vi "创建参数二维码.vi"() -> ()   [LabVIEW 2016, in "wxpusher.lvlib"]
uses:
  wxpusher.lvlib
  System.Windows.Forms
  <vilib>/Utility/miscctls.llb/LVPointTypeDef.ctl
  <vilib>/httpClient/POSTBuffer.vi
  <vilib>/httpClient/LabVIEWHTTPClient.lvlib
panel:
  out "url":string
  out "data.uid":string
  in  "测试":bool
  out "关注时间":string
  in  "关注信息":refnum<k24>(container) caption="黎山萧"
  in  "关闭":bool
  in  "带参数二维码":refnum<k24>(container)
  out "error out":errorcluster caption="错误输出"
  in  "error in (no error)":errorcluster caption="错误输入（无错误）"
  # "请使用微信扫描以下二维码"
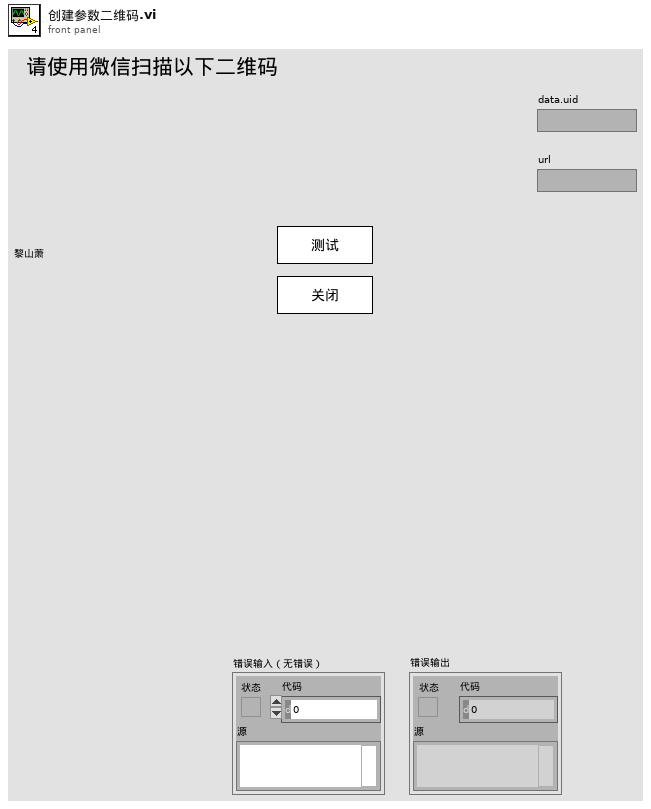
[diagram p1: front panel]
types:
  T1 = enum16{"初始化", "创建带参数二维码", "与服务器创建连接", "定时发送特征码", "接收回调信息", "处理回调信息", "展示关注信息", "结束"}[]
  T2 = enum16{"初始化", "创建带参数二维码", "与服务器创建连接", "定时发送特征码", "接收回调信息", "处理回调信息", "展示关注信息", "结束"}
  T3 = typedef "LVPointTypeDef.ctl" = cluster{"Horizontal":i16, "Vertical":i16}
  T4 = cluster{"code":u64, "msg":string, "data":cluster{"expires":u64, "code":string, "shortUrl":string, "extra":string, "url":string}, "success":bool}
  T5 = cluster{"appToken":string, "extra":string, "validTime":i32}
  T6 = enum16{"Standard", "Buffered", "CRLF", "Immediate"}
  T7 = cluster{"data":cluster{"action":string, "data":cluster{"appKey":string, "appName":string, "source":string, "time":u64, "uid":string, "userHeadImg":string, "userName":string, "extra":string}}}
  T8 = cluster{"cmd":string, "data":cluster{"png":u8[]}}
  T9 = typedef "LabVIEWHTTPClient.lvlib/ClientHandle.ctl" = refnum<k1>
  T10 = cluster{"expires":u64, "code":string, "shortUrl":string, "extra":string, "url":string}
  T11 = cluster{"action":string, "data":cluster{"appKey":string, "appName":string, "source":string, "time":u64, "uid":string, "userHeadImg":string, "userName":string, "extra":string}}
  T12 = cluster{"action":string, "data":cluster{"appKey":string, "appName":string, "source":string, "time":u64, "uid":string, "userHeadImg":string, "userName":string, "extra":string}}[]
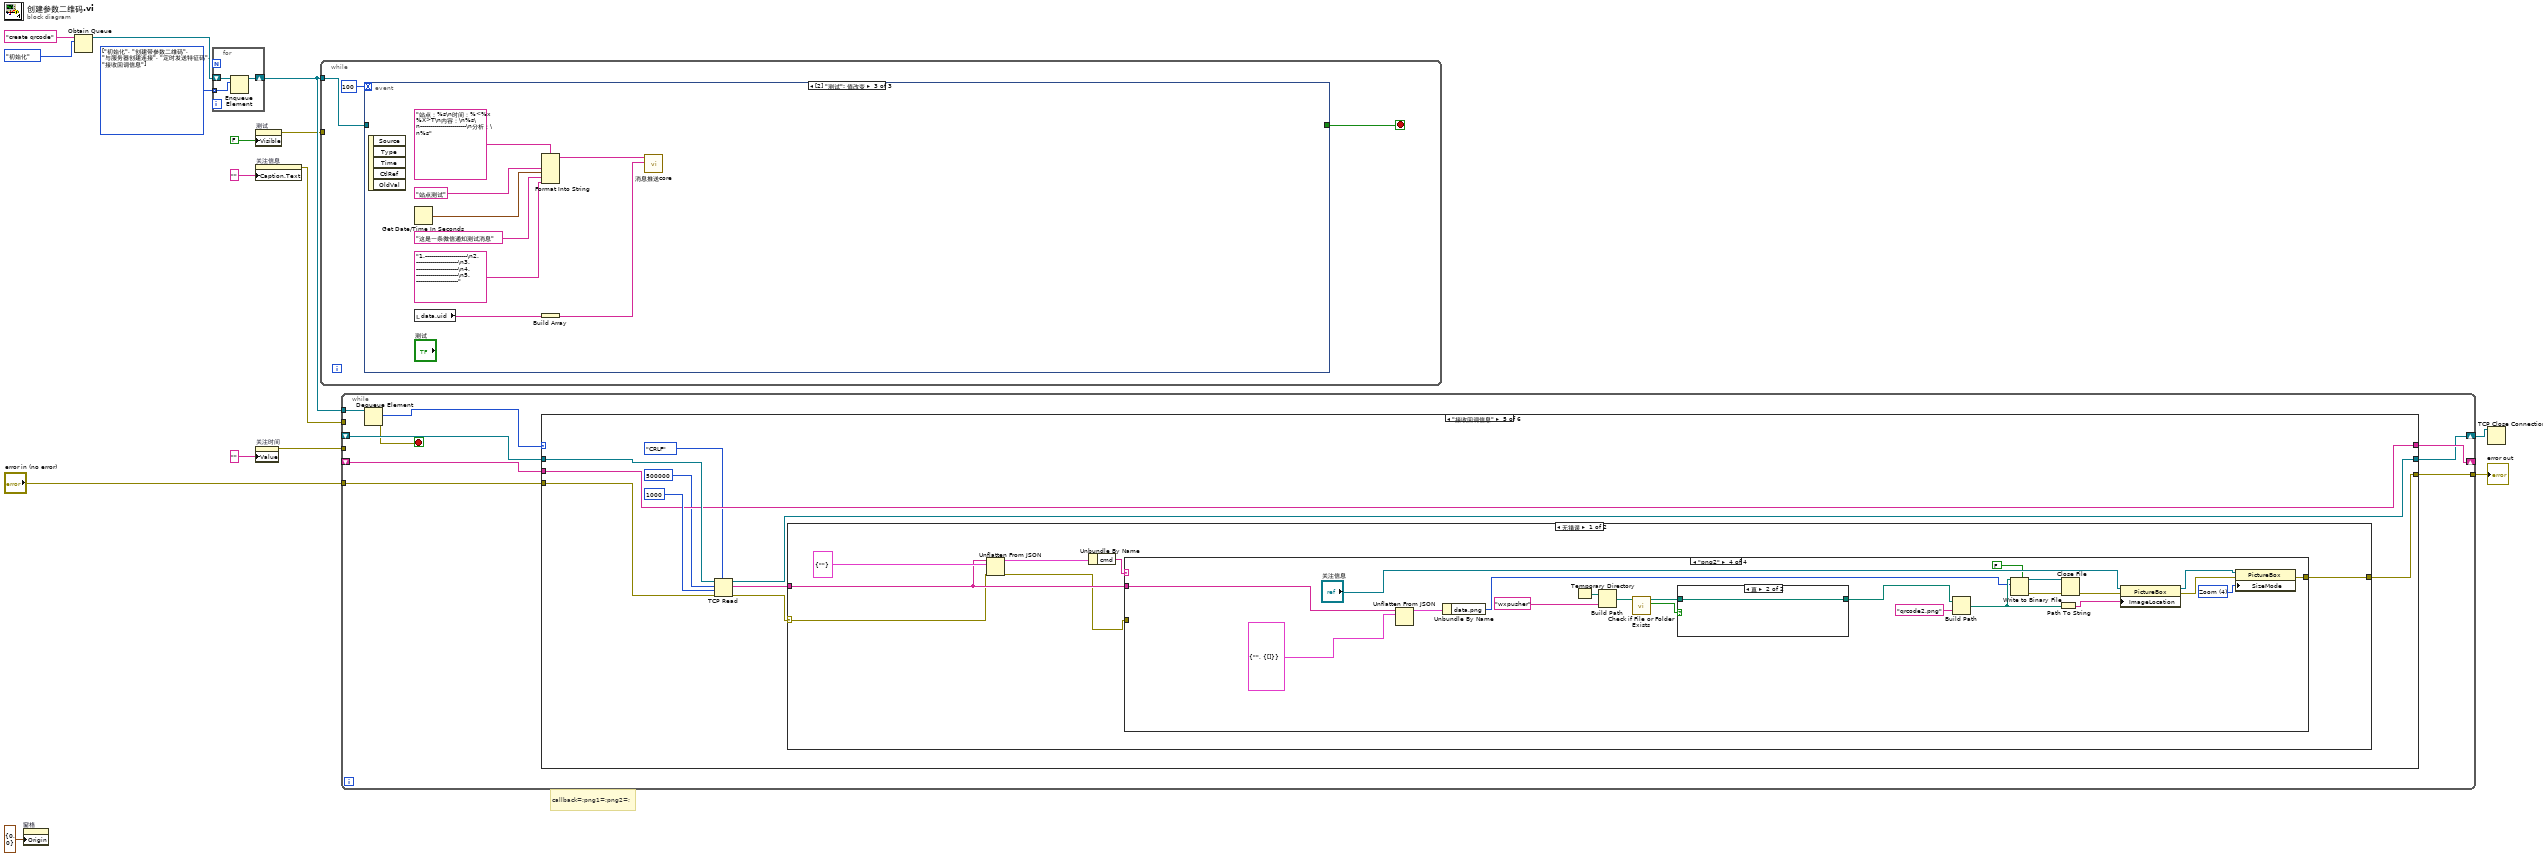
[diagram p0: block diagram]
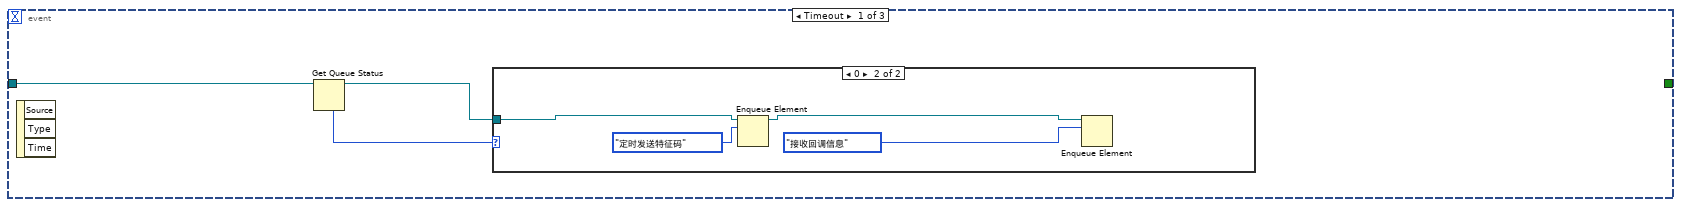
[diagram p2: hidden frame]
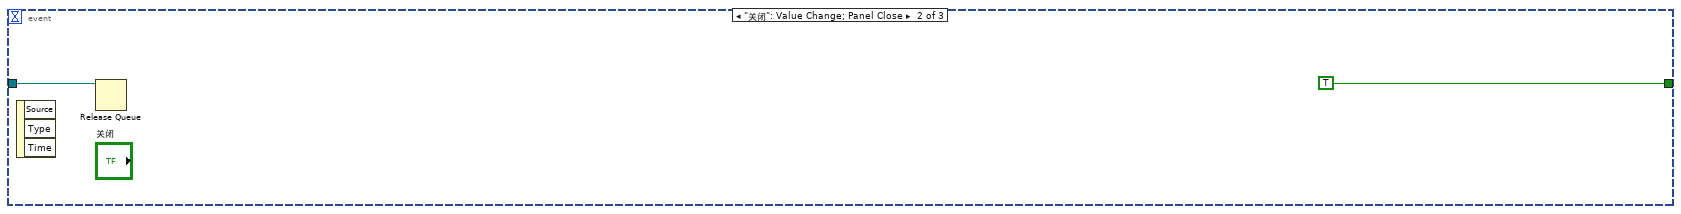
[diagram p4: hidden frame]
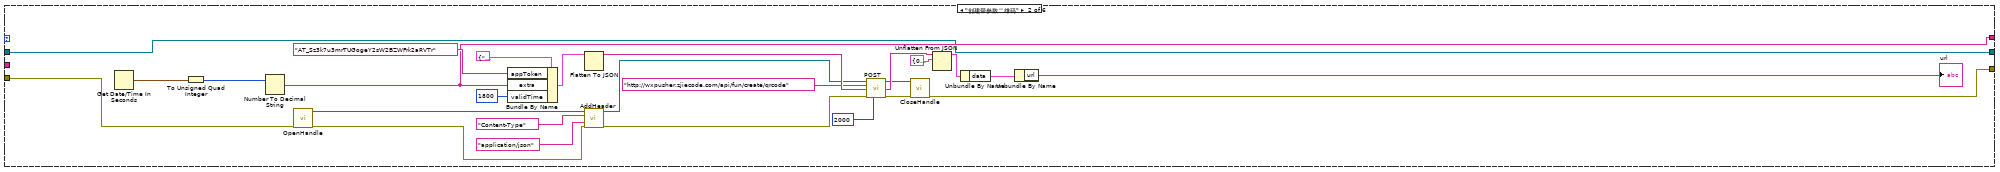
[diagram p6: hidden frame]
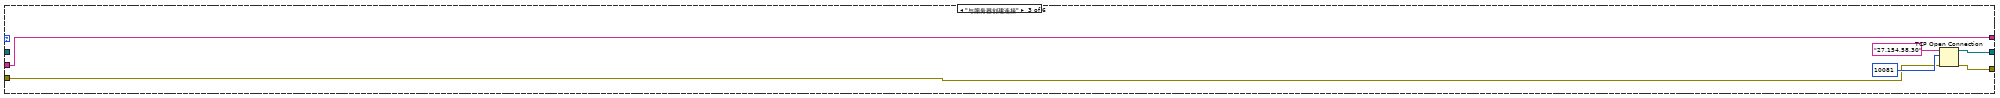
[diagram p7: hidden frame]
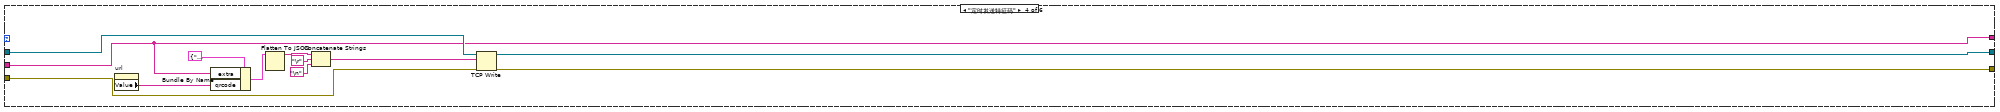
[diagram p8: hidden frame]
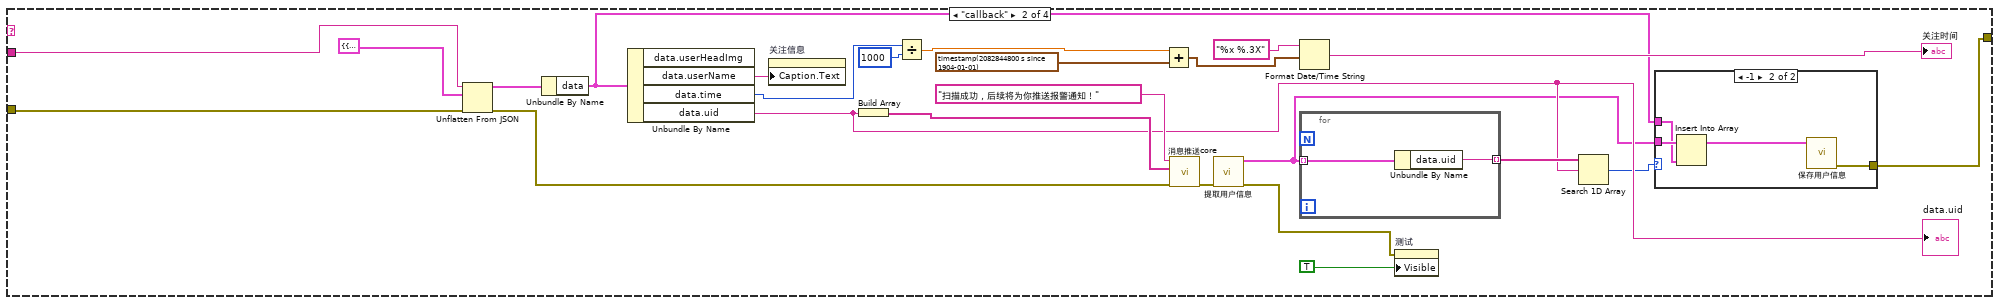
[diagram p10: hidden frame]
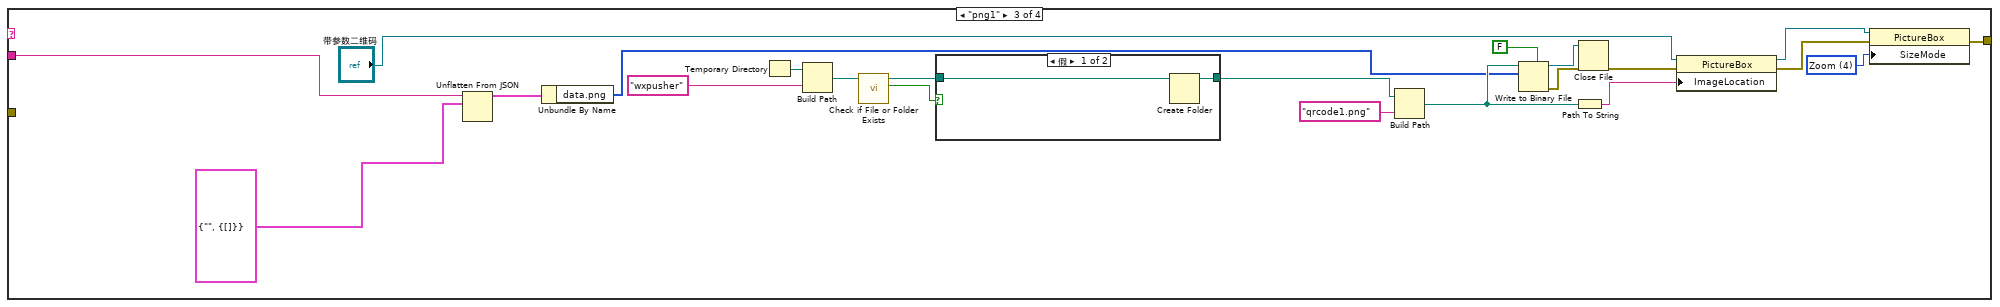
[diagram p12: hidden frame]
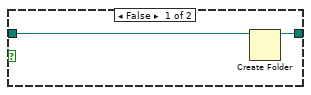
[diagram p14: hidden frame]
diagram:
  w8 = T1 [enum."初始化", enum."创建带参数二维码", enum."与服务器创建连接", enum."定时发送特征码", enum."接收回调信息"] items=["初始化", "创建带参数二维码", "与服务器创建连接", "定时发送特征码", "接收回调信息", "处理回调信息", "展示关注信息", "结束"]
  # "callback=;png1=;png2=;"
  n1 = property on="窗格" class="Pane"("Origin"=T3 {"Horizontal"=0, "Vertical"=0} ("原点")) -> ()  [unwired: 2 in, 2 out]
  n2 = Obtain Queue(name (unnamed)="create qrcode" ("名称（未命名）"), element data type=T2."初始化" ("枚举")) -> (queue out=w10:refnum<queue>)  [unwired: 3 in, 2 out]
  n3 = for {
    shift-right: [w17] -> w9
    shift-left: w10 -> [w18]
    tunnel: w8 -> [w16] mode=indexing
    n4 = Enqueue Element(queue=w18, element=w16) -> (queue out=w17:refnum<queue>)  [unwired: 2 in, 2 out]
  }
  n5 = property on="测试" class="Bool"("Visible"=FALSE ("可见")) -> (error out=w1:errorcluster)  [unwired: 2 in, 1 out]
  n6 = property on="关注信息" class="AXCont"("Caption.Text"="" ("标题.文本")) -> (error out=w7:errorcluster)  [unwired: 2 in, 1 out]
  n7 = property on="关注时间" class="Str"("Value"="" ("关注时间")) -> (error out=w5:errorcluster)  [unwired: 2 in, 1 out]
  n8 = while {
    tunnel: w9 -> [w20]
    tunnel: w1 -> [_]
    stop <- w21 stop-if-true
    n9 = event shown="[2] \"测试\": 值改变" {
      selector: _ -> [_ _ _]
      dyn-events: _ -> [_ _ _]
      timeout: 100 -> [_ _ _]
      tunnel: [_ TRUE _] -> w21
      tunnel: w20 -> [w24 w29 _]
      event Timeout {
        n10 = event-data() -> ()  [unwired: 1 in, 3 out]
        n11 = Get Queue Status(queue=w24) -> (queue out=w23:refnum<queue>, # elements in queue=w22:i32)  [unwired: 2 in, 6 out]
        n12 = case shown="0" w22 {
          tunnel: w23 -> [_ w25]
          frame Default {
          }
          frame 0 {
            n13 = Enqueue Element(queue=w25, element=T2."定时发送特征码" ("元素")) -> (queue out=w27:refnum<queue>)  [unwired: 2 in, 2 out]
            n14 = Enqueue Element(queue=w27, element=T2."接收回调信息" ("元素")) -> ()  [unwired: 2 in, 3 out]
          }
        }
      }
      event "关闭": Value Change; Panel Close {
        n15 = event-data() -> ()  [unwired: 1 in, 3 out]
        n16 = Release Queue(queue=w29) -> ()  [unwired: 2 in, 3 out]
      }
      event "测试": Value Change {
        n17 = event-data() -> ()  [unwired: 1 in, 5 out]
        n18 = Get Date/Time In Seconds() -> (seconds since 1Jan1904=w32:timestamp)
        n19 = local read "data.uid"() -> (w34:string)
        n20 = Format Into String(format string="站点：%s\n时间：%<%x %X>T\n内容：\n%s\n-----------------------\n分析：\n%s" ("格式字符串"), "站点测试" ("站点"), w32, "这是一条微信通知测试消息" ("内容"), "1.---------------------\n2.---------------------\n3.---------------------\n4.---------------------\n5.---------------------" ("分析")) -> (resulting string=w33:string)  [unwired: 2 in, 1 out]
        n21 = Build Array(w34) -> (w35:string[])
        n22 = call "消息推送core.vi"("数组"=w35, "content"=w33) -> ()  [unwired: 8 in, 2 out]
      }
    }
  }
  n23 = while {
    shift-right: [w47] -> _
    shift-left: _ -> [w46]
    tunnel: w9 -> [w45]
    tunnel: [w42] -> w12
    shift-right: [w43] -> w3
    shift-left: _ -> [w41]
    tunnel: "error in (no error)" -> [w40]
    tunnel: w7 -> [_]
    tunnel: w5 -> [_]
    stop <- w39 stop-if-true
    n24 = Dequeue Element(queue=w45) -> (element=w44:T2, error out=w39:errorcluster)  [unwired: 2 in, 2 out]
    n25 = case shown="\"接收回调信息\"" w44 {
      tunnel: [w50 w58 w79 w89 w100 w193] -> w47
      tunnel: w46 -> [w50 _ w79 w89 w100 w193]
      tunnel: [w49 w57 w80 w94 w101 w192] -> w43
      tunnel: [w48 w51 w78 w93 w98 _] -> w42
      tunnel: w41 -> [w49 w57 _ w92 w102 w192]
      tunnel: w40 -> [w48 w56 w77 w91 w99 _]
      frame "初始化", Default {
      }
      frame "创建带参数二维码" {
        n26 = Get Date/Time In Seconds() -> (seconds since 1Jan1904=w73:timestamp)
        n27 = To Unsigned Quad Integer(1:w73) -> (0:w74:u64)
        n28 = Number To Decimal String(number=w74) -> (decimal integer string=w58:string)  [unwired: 1 in]
        n29 = call <vilib>:"OpenHandle.vi"("error in (no error)"=w56) -> ("client handle out"=w59:T9, "error out"=w61:errorcluster)  [unwired: 13 in]
        n30 = Bundle By Name(cluster=T5 {"appToken"="", "extra"="", "validTime"=0}, "appToken"="AT_Sz3k7u3mrTUGogeY2sW2BZWFrk2aRVTr", "extra"=w58, "validTime"=1800 ("contentType")) -> (w69:T5)
        n31 = Flatten To JSON(anything=w69) -> (JSON string=w70:string)  [unwired: 2 in, 1 out]
        n32 = call <vilib>:"AddHeader.vi"("client handle"=w59, "header"="Content-Type", "value"="application/json", "error in (no error)"=w61) -> ("client handle out"=w60:T9, "error out"=w64:errorcluster)  [unwired: 10 in]
        n33 = call-poly <vilib>:"POST.vi"("client handle"=w60, "url"="http://wxpusher.zjiecode.com/api/fun/create/qrcode", "buffer"=w70, "error in (no error)"=w64, "timeout (10000)"=2000) -> ("client handle out"=w52:T9, "body"=w71:string, "error out"=w53:errorcluster)  [unwired: 7 in, 1 out]
        n34 = call <vilib>:"CloseHandle.vi"("client handle"=w52, "error in (no error)"=w53) -> ("error out"=w51:errorcluster)  [unwired: 13 in]
        n35 = Unflatten From JSON(JSON string=w71, type and defaults=T4 {"code"=0, "msg"="", "data"={"expires"=0, "code"="", "shortUrl"="", "extra"="", "url"=""}, "success"=FALSE}) -> (value=w76:T4)  [unwired: 5 in, 1 out]
        n36 = Unbundle By Name(w76) -> ("data"=w75:T10)
        n37 = Unbundle By Name(w75) -> ("url"=→"url":string)
      }
      frame "与服务器创建连接" {
        n38 = TCP Open Connection(address="27.154.58.30" ("地址"), remote port or service name=u16 10081 ("远程端口或服务名称"), error in (no error)=w77) -> (connection ID=w80:refnum<k5>, error out=w78:errorcluster)  [unwired: 2 in]
      }
      frame "定时发送特征码" {
        n39 = property on="url" class="Str"() -> ("Value"=w88:string)  [unwired: 2 in, 2 out]
        n40 = Bundle By Name(cluster=cluster{"extra":string, "qrcode":string} {"extra"="", "qrcode"=""}, "extra"=w89, "qrcode"=w88) -> (w85:cluster{"extra":string, "qrcode":string})
        n41 = Flatten To JSON(anything=w85) -> (JSON string=w84:string)  [unwired: 2 in, 1 out]
        n42 = Concatenate Strings(w84, "\r", "\n") -> (w83:string)
        n43 = TCP Write(connection ID=w92, data in=w83, error in (no error)=w91) -> (connection ID out=w94:refnum<k5>, error out=w93:errorcluster)  [unwired: 1 in, 1 out]
      }
      frame "接收回调信息" {
        n44 = TCP Read(connection ID=w102, bytes to read=500000 ("读取的字节"), error in (no error)=w99, 7:T6."CRLF" ("模式（标准）"), 9:1000 ("超时毫秒(25000)")) -> (connection ID out=w101:refnum<k5>, data out=w104:string, error out=w96:errorcluster)
        n45 = case shown="无错误" w96 {
          selector: w96 -> [w106 _]
          tunnel: [w111 _] -> w98
          tunnel: w104 -> [w107 _]
          frame No Error {
            n46 = Unflatten From JSON(JSON string=w107, type and defaults=cluster{"cmd":string} {"cmd"=""}, error in (no error)=w106) -> (value=w109:cluster{"cmd":string}, error out=w105:errorcluster)  [unwired: 4 in]
            n47 = Unbundle By Name(w109) -> ("cmd"=w108:string)
            n48 = case shown="\"png2\"" w108 {
              tunnel: [_ w119 w147 w178] -> w111
              tunnel: w105 -> [_ w118 _ _]
              tunnel: w107 -> [_ w114 w145 w170]
              frame "假", Default {
              }
              frame "callback" {
                n49 = Unflatten From JSON(JSON string=w114, type and defaults=T7 {"data"={"action"="", "data"={"appKey"="", "appName"="", "source"="", "time"=0, "uid"="", "userHeadImg"="", "userName"="", "extra"=""}}} ("输出簇"), error in (no error)=w118) -> (value=w116:T7, error out=w127:errorcluster)  [unwired: 4 in]
                n50 = Unbundle By Name(w116) -> ("data"=w115:T11)
                n51 = Unbundle By Name(w115) -> ("data.userName"=w128:string, "data.time"=w135:u64, "data.uid"=w123:string)  [unwired: 1 out]
                "data.uid" <- w123
                n52 = property on="关注信息" class="AXCont"("Caption.Text"=w128) -> ()  [unwired: 2 in, 2 out]
                n53 = Build Array(w123) -> (w125:string[])
                n54 = Divide(x=w135, y=u64 1000) -> (x/y=w133:dbl)
                n55 = Add(x=w133, y=timestamp(2082844800 s since 1904-01-01)) -> (x+y=w131:timestamp)
                n56 = call "消息推送core.vi"("error in (no error)"=w127, "数组"=w125, "content"="扫描成功，后续将为你推送报警通知！") -> ("error out"=w120:errorcluster)  [unwired: 7 in, 1 out]
                n57 = call "提取用户信息.vi"("error in (no error)"=w120) -> ("error out"=w112:errorcluster, "用户信息"=w121:T12)  [unwired: 9 in]
                n58 = Format Date/Time String(time format string (%c)="%x %.3X" ("时间格式字符串(%c)"), seconds (now)=w131) -> (date/time string=→"关注时间":string)  [unwired: 1 in]
                n59 = for {
                  tunnel: w121 -> [w141] mode=indexing
                  tunnel: [w140] -> w124 mode=indexing
                  n60 = Unbundle By Name(w141) -> ("data.uid"=w140:string)
                }
                n61 = property on="测试" class="Bool"(error in=w112, "Visible"=TRUE ("可见")) -> ()  [unwired: 1 in, 2 out]
                n62 = Search 1D Array(1D array=w124, element=w123) -> (index of element=w122:i32)  [unwired: 1 in]
                n63 = case shown="-1" w122 {
                  tunnel: w121 -> [_ w139]
                  tunnel: w115 -> [_ w138]
                  tunnel: [_ w136] -> w119
                  frame 0, Default {
                  }
                  frame -1 {
                    n64 = Insert Into Array(array=w139, new element=w138) -> (w137:T12)  [unwired: 1 in]
                    n65 = call "保存用户信息.vi"("用户信息"=w137) -> ("error out"=w136:errorcluster)  [unwired: 10 in]
                  }
                }
              }
              frame "png1" {
                w154 = 4 items=["Normal", "StretchImage", "AutoSize", "CenterImage", "Zoom"] ("SizeMode")
                n66 = Unflatten From JSON(JSON string=w145, type and defaults=T8 {"cmd"="", "data"={"png"=[]}}) -> (value=w144:T8)  [unwired: 5 in, 1 out]
                n67 = Unbundle By Name(w144) -> ("data.png"=w143:u8[])
                n68 = Temporary Directory() -> (w163:path)
                n69 = Build Path(base path=w163, name or relative path="wxpusher" ("名称或相对路径")) -> (appended path=w158:path)
                n70 = call <vilib>:"Check if File or Folder Exists.vi"("path"=w158) -> ("file or folder exists?"=w161:bool, "dup path"=w160:path)  [unwired: 8 in, 1 out]
                n71 = case shown="假" w161 {
                  tunnel: [w164 w166] -> w157
                  tunnel: w160 -> [w165 w166]
                  frame False {
                    n72 = Create Folder(path (use dialog)=w165) -> (created path=w164:path)  [unwired: 2 in, 2 out]
                  }
                  frame True {
                  }
                }
                n73 = Build Path(base path=w157, name or relative path="qrcode1.png" ("名称或相对路径")) -> (appended path=w149:path)
                n74 = Write to Binary File(file (use dialog)=w149, data=w143, 5:FALSE ("预置数组或字符串大小？ (T)")) -> (refnum out=w156:refnum<file>, error out=w155:errorcluster)  [unwired: 3 in, 1 out]
                n75 = Path To String(path=w149) -> (string=w150:string)
                n76 = Close File(refnum=w156, error in=w155) -> (error out=w148:errorcluster)  [unwired: 1 out]
                n77 = property on="属性节点" class="PictureBox"(reference="带参数二维码", error in=w148, "ImageLocation"=w150) -> (reference out=w153:refnum<k24>, error out=w151:errorcluster)
                n78 = property class="PictureBox"(reference=w153, error in=w151, "SizeMode"=w154) -> (error out=w147:errorcluster)  [unwired: 1 out]
              }
              frame "png2" {
                w186 = 4 items=["Normal", "StretchImage", "AutoSize", "CenterImage", "Zoom"] ("SizeMode")
                n79 = Unflatten From JSON(JSON string=w170, type and defaults=T8 {"cmd"="", "data"={"png"=[]}}) -> (value=w171:T8)  [unwired: 5 in, 1 out]
                n80 = Unbundle By Name(w171) -> ("data.png"=w169:u8[])
                n81 = Temporary Directory() -> (w177:path)
                n82 = Build Path(base path=w177, name or relative path="wxpusher" ("名称或相对路径")) -> (appended path=w173:path)
                n83 = call <vilib>:"Check if File or Folder Exists.vi"("path"=w173) -> ("file or folder exists?"=w175:bool, "dup path"=w174:path)  [unwired: 8 in, 1 out]
                n84 = case shown="真" w175 {
                  tunnel: [w189 w191] -> w172
                  tunnel: w174 -> [w190 w191]
                  frame False {
                    n85 = Create Folder(path (use dialog)=w190) -> (created path=w189:path)  [unwired: 2 in, 2 out]
                  }
                  frame True {
                  }
                }
                n86 = Build Path(base path=w172, name or relative path="qrcode2.png" ("名称或相对路径")) -> (appended path=w180:path)
                n87 = Write to Binary File(file (use dialog)=w180, data=w169, 5:FALSE ("预置数组或字符串大小？ (T)")) -> (refnum out=w183:refnum<file>, error out=w184:errorcluster)  [unwired: 3 in, 1 out]
                n88 = Path To String(path=w180) -> (string=w179:string)
                n89 = Close File(refnum=w183, error in=w184) -> (error out=w182:errorcluster)  [unwired: 1 out]
                n90 = property on="属性节点" class="PictureBox"(reference="关注信息", error in=w182, "ImageLocation"=w179) -> (reference out=w187:refnum<k24>, error out=w181:errorcluster)
                n91 = property class="PictureBox"(reference=w187, error in=w181, "SizeMode"=w186) -> (error out=w178:errorcluster)  [unwired: 1 out]
              }
            }
          }
          frame Error {
          }
        }
      }
      frame "结束" {
      }
    }
  }
  "error out" <- w12
  n92 = TCP Close Connection(connection ID=w3) -> ()  [unwired: 2 in, 2 out]
